vi "Update All Values.vi"(8 "error in (no error)":errorcluster, 10 "Values":refnum<class "Type.lvclass">[](array[class]), 11 "Long Class Name Entity Example in":refnum<class "Long Class Name Entity Example.lvclass">) -> (0 "error out":errorcluster, 3 "Long Class Name Entity Example out":refnum<class "Long Class Name Entity Example.lvclass">)   [LabVIEW 2022 SP3, in "Conditum-Example.lvlib" / "Long Class Name Entity Example.lvclass"]
uses:
  Long Class Name Entity Example.lvclass
  Conditum/Columns/Type/Type.lvclass
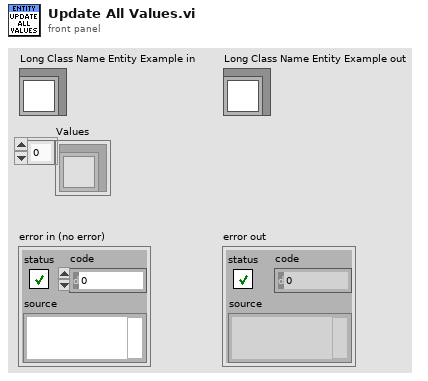
[diagram p1: front panel]
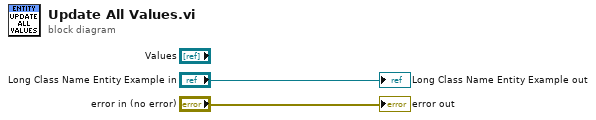
[diagram p0: block diagram]
diagram:
  "error out" <- "error in (no error)"
  "Long Class Name Entity Example out" <- "Long Class Name Entity Example in"
